vi "Write Optional Plane Labels.vi"(5 "Optional Plane Labels":bool, 9 "XYGraph in":refnum<class "XYGraph.lvclass">) -> (3 "XYGraph out":refnum<class "XYGraph.lvclass">)   [LabVIEW 2014, in "XYGraph.lvclass"]
uses:
  XYGraph.lvclass
  XYGraph.lvclass/XYGraph.ctl
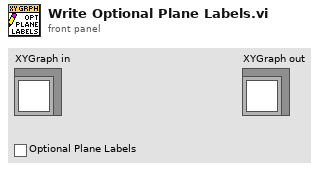
[diagram p1: front panel]
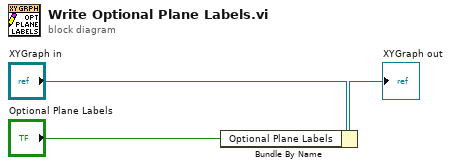
[diagram p0: block diagram]
diagram:
  n1 = Bundle By Name(cluster="XYGraph in", "Optional Plane Labels"="Optional Plane Labels") -> (→"XYGraph out":refnum<class "XYGraph.lvclass">)
